vi "GetRobotPosition.vi"(8 "error in (no error)":errorcluster, 11 "Robot_Interface in":refnum<class "Robot_Interface.lvclass">) -> (0 "error out":errorcluster, 2 "Robot Position":T1={"Claw"=0.5192802056555269, "JointA"=347.1752980785341, "JointB"=280.93136534375475, "JointC"=30.749358432304007, "JointD"=30.749358432304007}, 3 "Robot_Interface out":refnum<class "Robot_Interface.lvclass">)   [LabVIEW 2015, in "Robot_Interface.lvclass"]
uses:
  Robot_Interface.lvclass
  Subsytems/JKI.Robot.SMO/Typedefs/RobotPosition--Cluster.ctl
  Robot_Interface.lvclass/Robot_Interface.ctl
  Subsytems/JKI.Robot.SMO.Base/JKI.Robot.SMO.Base.lvclass
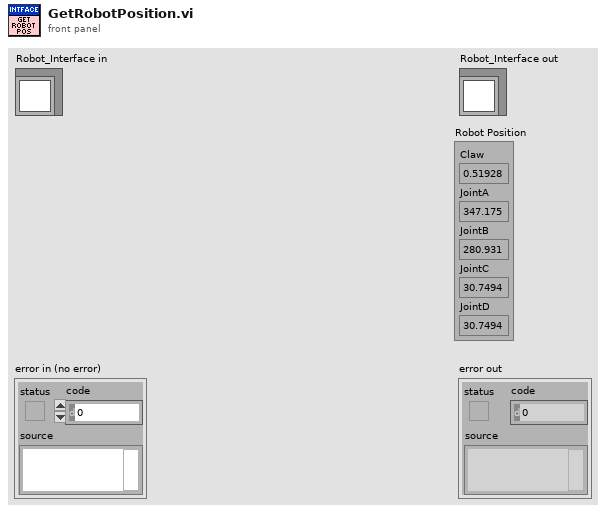
[diagram p1: front panel]
types:
  T1 = typedef "RobotPosition--Cluster.ctl" = cluster{"Claw":dbl, "JointA":dbl, "JointB":dbl, "JointC":dbl, "JointD":dbl}
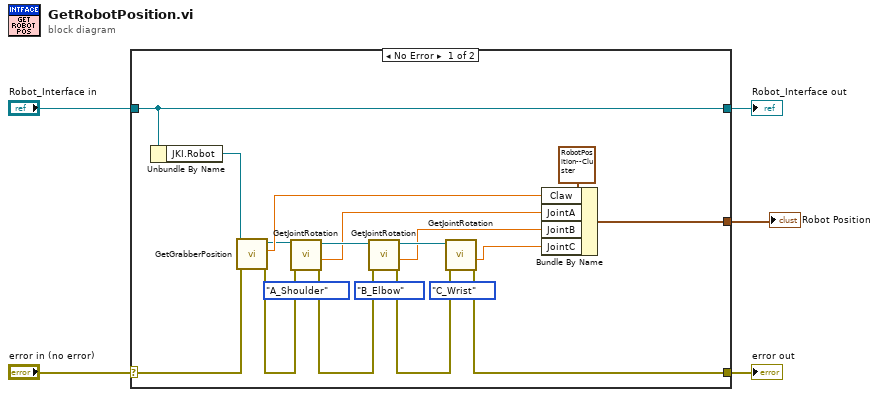
[diagram p0: block diagram]
diagram:
  n1 = case shown="No Error" "error in (no error)" {
    selector: "error in (no error)" -> [w7 w26]
    tunnel: [w6 w26] -> w4
    tunnel: [w9 w25] -> w2
    tunnel: "Robot_Interface in" -> [w9 w25]
    tunnel: [w10 _] -> w1
    frame No Error {
      n2 = Unbundle By Name(w9) -> ("JKI.Robot"=w8:refnum<class "JKI.Robot.SMO.Base.lvclass">)
      n3 = call-dynamic "GetGrabberPosition.vi"("error in (no error)"=w7, "JKI.Robot.SMO.Base.lvclass"=w8) -> ("error out"=w22:errorcluster, "SetGrabberPosition"=w16:dbl, "JKI.Robot.SMO.Base.lvclass"=w11:refnum<class "JKI.Robot.SMO.Base.lvclass">)  [unwired: 7 in]
      n4 = call-dynamic "GetJointRotation.vi"("error in (no error)"=w22, "Joint"=enum16{"A_Shoulder", "B_Elbow", "C_Wrist"}."A_Shoulder" ("JointType"), "JKI.Robot.SMO.Base"=w11) -> ("error out"=w23:errorcluster, "Rotation (Deg)"=w17:dbl, "JKI.Robot.SMO.Base"=w20:refnum<class "JKI.Robot.SMO.Base.lvclass">)  [unwired: 6 in]
      n5 = call-dynamic "GetJointRotation.vi"("error in (no error)"=w23, "Joint"=enum16{"A_Shoulder", "B_Elbow", "C_Wrist"}."B_Elbow" ("JointType"), "JKI.Robot.SMO.Base"=w20) -> ("error out"=w24:errorcluster, "Rotation (Deg)"=w18:dbl, "JKI.Robot.SMO.Base"=w21:refnum<class "JKI.Robot.SMO.Base.lvclass">)  [unwired: 6 in]
      n6 = call-dynamic "GetJointRotation.vi"("error in (no error)"=w24, "Joint"=enum16{"A_Shoulder", "B_Elbow", "C_Wrist"}."C_Wrist" ("JointType"), "JKI.Robot.SMO.Base"=w21) -> ("error out"=w6:errorcluster, "Rotation (Deg)"=w19:dbl)  [unwired: 6 in, 1 out]
      n7 = Bundle By Name(cluster=T1 {"Claw"=0.5192802056555269, "JointA"=347.1752980785341, "JointB"=280.93136534375475, "JointC"=30.749358432304007, "JointD"=30.749358432304007} ("Robot Position"), "Claw"=w16, "JointA"=w17, "JointB"=w18, "JointC"=w19) -> (w10:T1)
    }
    frame Error {
    }
  }
  "error out" <- w4
  "Robot_Interface out" <- w2
  "Robot Position" <- w1
